vi "禹山浊度_获取温度和测量值.vi"(8 "error in (no error)":errorcluster caption="错误输入（无错误）", 11 "MB_Serial session in":refnum<class "MB_Master_Serial.lvclass">) -> (0 "error out":errorcluster caption="错误输出", 2 "输出值":cluster{"温度测量值":sgl, "浊度":sgl}, 3 "MB_Serial session out":refnum<class "MB_Master_Serial.lvclass">)   [LabVIEW 2016, in "斯坦道多参数.lvlib"]
uses:
  <vilib>/Plasmionique/MB Master/MB_Master_Serial/MB_Master_Serial.lvclass
  C:/Program Files (x86)/National Instruments/LabVIEW 2016/vi.lib/Plasmionique/MB Master/MB_Master/MB_Master.lvclass
  <vilib>/Plasmionique/MB Master/MB Master.lvlib
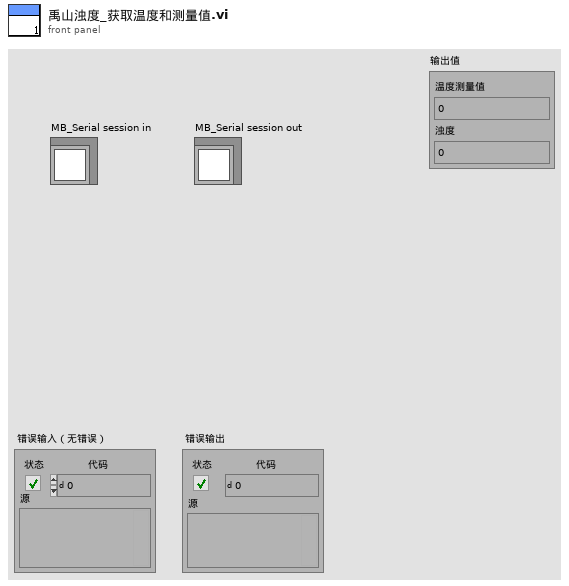
[diagram p1: front panel]
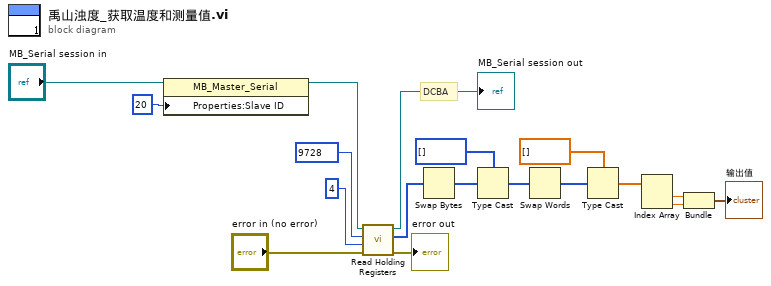
[diagram p0: block diagram]
diagram:
  # "DCBA"
  n1 = property class="MB_Master_Serial"(reference="MB_Serial session in", "Properties:Slave ID"=u16 20 ("y")) -> (reference out=w9:refnum<class "MB_Master_Serial.lvclass">)  [unwired: 1 in, 1 out]
  n2 = call <vilib>:"Read Holding Registers.vi"("error in (no error)"="error in (no error)", "quantity"=u16 4, "starting address"=u16 9728, "MB session in"=w9) -> ("error out"=→"error out":errorcluster, "Registers"=w4:u16[], "MB session out"=→"MB_Serial session out":refnum<class "MB_Master_Serial.lvclass">)  [unwired: 5 in]
  n3 = Swap Bytes(anything=w4) -> (byte swapped=w3:u16[])
  n4 = Type Cast(type=u32[] [] ("数组 2"), x=w3) -> (*(type *) &x=w13:u32[])
  n5 = Swap Words(1:w13) -> (0:w15:u32[])
  n6 = Type Cast(type=sgl[] [] ("数组 2"), x=w15) -> (*(type *) &x=w11:sgl[])
  n7 = Index Array(array=w11) -> (element #1=w2:sgl, element #2=w1:sgl)  [unwired: 2 in]
  n8 = Bundle("数值"=w2, "数值"=w1) -> (→"输出值":cluster{"数值":sgl, "数值":sgl})  [unwired: 1 in]
